vi "FX_Config_Set Output Values.vi"(6 "Send Cmd Timout(ms)":u32, 8 "Error":errorcluster, 9 "Output":T6 {"Min"."REV" format="%.2f"; "Min"."FWD" format="%.2f"; "Max"."REV" format="%.2f"; "Max"."FWD" format="%.2f"}, 11 "PhoenixMotorControlDevRef":T1) -> (0 "Error Out":errorcluster, 3 "PhoenixMotorControlDevRef Out":T1)   [LabVIEW 2023]
uses:
  Shared Code/TypeDefs/Cluster_Config FX Motor Output.ctl
  <vilib>/Rock Robotics/WPI/ThirdParty/Phoenix-LabVIEW/Motor Controller/Controls/CTRE_Phoenix_MotorControl_TalonFXInvertType.ctl
  <vilib>/Rock Robotics/WPI/ThirdParty/Phoenix-LabVIEW/Motor Controller/Controls/CTRE_Phoenix_MotorControl_NeutralMode.ctl
  Shared Code/TypeDefs/Cluster_FWD  REV Values.ctl
  <vilib>/Rock Robotics/WPI/MotorControl/WPI_MotorControlDeviceRef.ctl
  <vilib>/Rock Robotics/WPI/MotorControl/WPI_MotorControlType.ctl
  <vilib>/Rock Robotics/SystemInterfaces/DIO/FPGA_DIOPWMChannel.ctl
  <vilib>/Rock Robotics/WPI/PWM/WPI_PWMDeadband.ctl
  <vilib>/Rock Robotics/SystemInterfaces/DIO/FPGA_DIOChannel.ctl
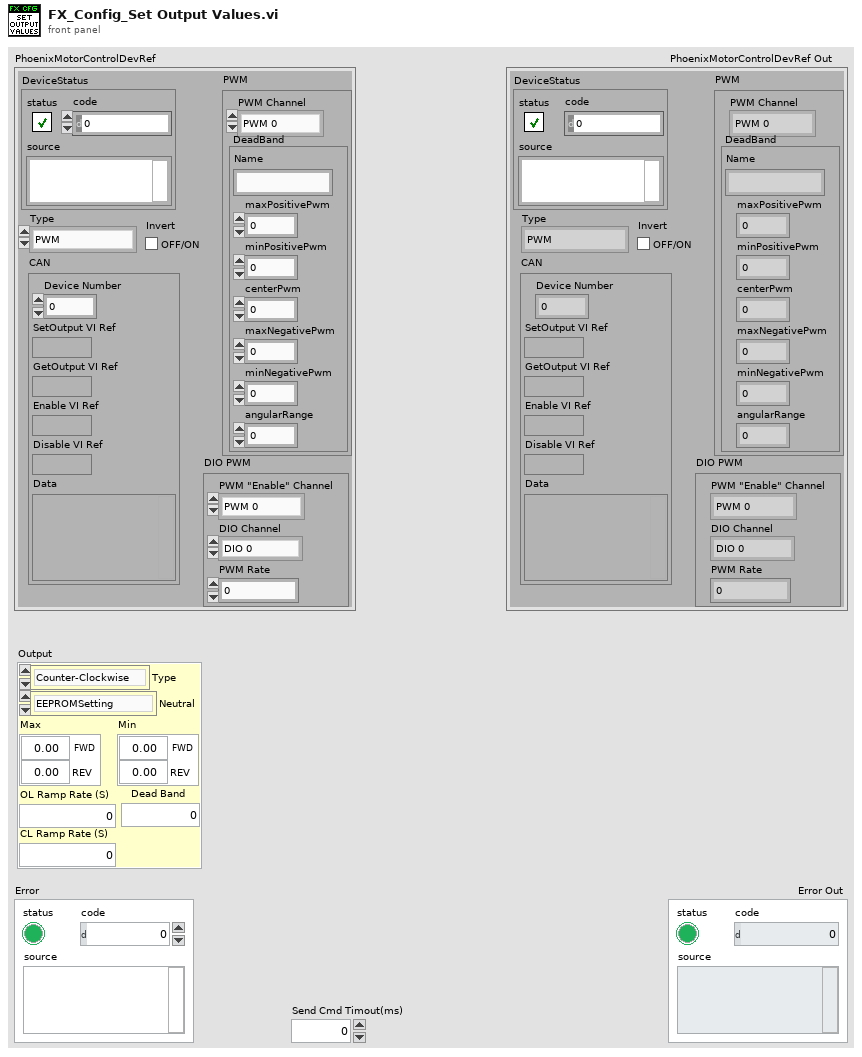
[diagram p1: front panel]
types:
  T1 = typedef "WPI_MotorControlDeviceRef.ctl" = cluster{"DeviceStatus":errorcluster, "Type":T2, "PWM":cluster{"PWM Channel":T3, "DeadBand":T4}, "CAN":cluster{"Device Number":u8, "SetOutput VI Ref":variant, "GetOutput VI Ref":variant, "Enable VI Ref":variant, "Disable VI Ref":variant, "Data":variant}, "Invert":bool, "DIO PWM":cluster{"PWM \"Enable\" Channel":T3, "DIOChannel":T5, "PWM Rate":dbl}}
  T2 = typedef "WPI_MotorControlType.ctl" = enum16{"PWM", "CAN", "DIO PWM"}
  T3 = typedef "FPGA_DIOPWMChannel.ctl" = enum8{"PWM 0", "PWM 1", "PWM 2", "PWM 3", "PWM 4", "PWM 5", "PWM 6", "PWM 7", "PWM 8", "PWM 9", "PWM MXP 0", "PWM MXP 1", "PWM MXP 2", "PWM MXP 3", "PWM MXP 4", "PWM MXP 5", "PWM MXP 6", "PWM MXP 7", "PWM MXP 8", "PWM MXP 9", "Invalid"}
  T4 = typedef "WPI_PWMDeadband.ctl" = cluster{"Name":string, "maxPositivePwm":i32, "minPositivePwm":i32, "centerPwm":i32, "maxNegativePwm":i32, "minNegativePwm":i32, "angularRange":u16}
  T5 = typedef "FPGA_DIOChannel.ctl" = enum8{"DIO 0", "DIO 1", "DIO 2", "DIO 3", "DIO 4", "DIO 5", "DIO 6", "DIO 7", "DIO 8", "DIO 9", "DIO MXP 0", "DIO MXP 1", "DIO MXP 2", "DIO MXP 3", "DIO MXP 4", "DIO MXP 5", "DIO MXP 6", "DIO MXP 7", "DIO MXP 8", "DIO MXP 9", "DIO MXP 10", "DIO MXP 11", "DIO MXP 12", "DIO MXP 13", "DIO MXP 14", "DIO MXP 15", "SPI Port CS1", "SPI Port CS2", "SPI Port CS3", "SPI Port MISO", "SPI Port MOSI", "Invalid"}
  T6 = typedef "Cluster_Config FX Motor Output.ctl" = cluster{"Type":T7, "Neutral":T8, "Max":T9, "Min":T9, "OL Ramp Rate (S)":dbl, "Dead Band":dbl, "CL Ramp Rate (S)":dbl}
  T7 = typedef "CTRE_Phoenix_MotorControl_TalonFXInvertType.ctl" = enum16{"Counter-Clockwise", "Clockwise"}
  T8 = typedef "CTRE_Phoenix_MotorControl_NeutralMode.ctl" = enum8{"EEPROMSetting", "Override to Coast", "Override to Brake"}
  T9 = typedef "Cluster_FWD  REV Values.ctl" = cluster{"FWD":dbl, "REV":dbl}
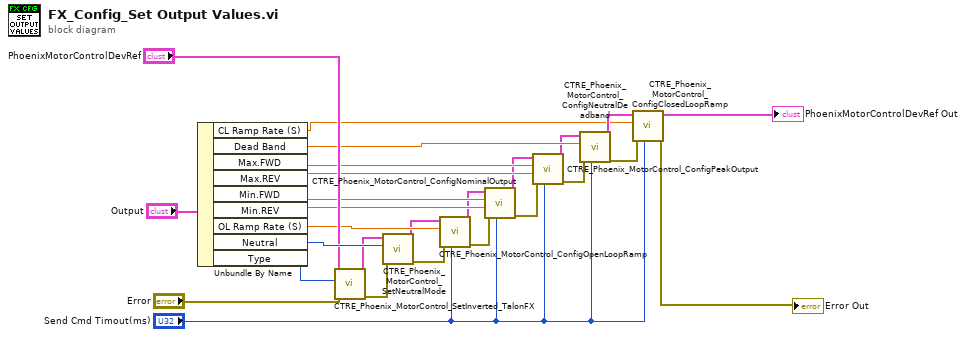
[diagram p0: block diagram]
diagram:
  n1 = Unbundle By Name("Output") -> ("CL Ramp Rate (S)"=w4:dbl, "Dead Band"=w12:dbl, "Max.FWD"=w15:dbl, "Max.REV"=w16:dbl, "Min.FWD"=w19:dbl, "Min.REV"=w20:dbl, "OL Ramp Rate (S)"=w23:dbl, "Neutral"=w25:T8, "Type"=w26:T7)
  n2 = call <vilib>:"CTRE_Phoenix_MotorControl_SetInverted_TalonFX.vi"("error in (no error)"="Error", "Invert Type"=w26, "PhoenixMotorControlDevRef"="PhoenixMotorControlDevRef") -> ("error out"=w8:errorcluster, "PhoenixMotorControlDevRef"=w7:T1)  [unwired: 7 in]
  n3 = call <vilib>:"CTRE_Phoenix_MotorControl_SetNeutralMode.vi"("error in (no error)"=w8, "Motor Control Neutral Mode"=w25, "PhoenixMotorControlDevRef"=w7) -> ("error out"=w21:errorcluster, "PhoenixMotorControlDevRef"=w22:T1)  [unwired: 7 in]
  n4 = call <vilib>:"CTRE_Phoenix_MotorControl_ConfigOpenLoopRamp.vi"("timeoutMs"="Send Cmd Timout(ms)", "error in (no error)"=w21, "secondsFromNeutralToFull"=w23, "PhoenixMotorControlDevRef"=w22) -> ("error out"=w17:errorcluster, "PhoenixMotorControlDevRef"=w18:T1)  [unwired: 6 in]
  n5 = call <vilib>:"CTRE_Phoenix_MotorControl_ConfigNominalOutput.vi"("timeoutMs"="Send Cmd Timout(ms)", "error in (no error)"=w17, "Reverse Nominal Percent Output"=w20, "Forward Nominal Percent Output"=w19, "PhoenixMotorControlDevRef"=w18) -> ("error out"=w13:errorcluster, "PhoenixMotorControlDevRef"=w14:T1)  [unwired: 5 in]
  n6 = call <vilib>:"CTRE_Phoenix_MotorControl_ConfigPeakOutput.vi"("timeoutMs"="Send Cmd Timout(ms)", "error in (no error)"=w13, "Reverse Peak Percent Output"=w16, "Forward Peak Percent Output"=w15, "PhoenixMotorControlDevRef"=w14) -> ("error out"=w10:errorcluster, "PhoenixMotorControlDevRef"=w11:T1)  [unwired: 5 in]
  n7 = call <vilib>:"CTRE_Phoenix_MotorControl_ConfigNeutralDeadband.vi"("timeoutMs"="Send Cmd Timout(ms)", "error in (no error)"=w10, "Percent Deadband"=w12, "PhoenixMotorControlDevRef"=w11) -> ("error out"=w3:errorcluster, "PhoenixMotorControlDevRef"=w6:T1)  [unwired: 6 in]
  n8 = call <vilib>:"CTRE_Phoenix_MotorControl_ConfigClosedLoopRamp.vi"("timeoutMs"="Send Cmd Timout(ms)", "error in (no error)"=w3, "secondsFromNeutralToFull"=w4, "PhoenixMotorControlDevRef"=w6) -> ("error out"=→"Error Out":errorcluster, "PhoenixMotorControlDevRef"=→"PhoenixMotorControlDevRef Out":T1)  [unwired: 6 in]
